vi "setfilter.vi"(2 "error in (no error)":errorcluster, 3 "Filter":i32=1 min=1 max=6 step=1) -> (0 "error out":errorcluster)   [LabVIEW 2017]
doc: "Selects the filter for monochromator to use"
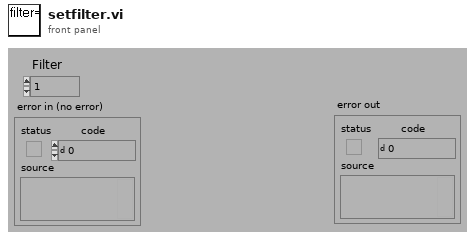
[diagram p1: front panel]
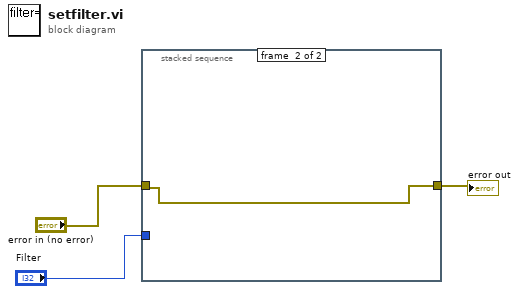
[diagram p0: block diagram]
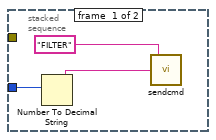
[diagram p2: hidden frame]
diagram:
  n1 = stacked-sequence {
    tunnel: "error in (no error)" -> [_ w7]
    tunnel: [_ w7] -> w2
    tunnel: "Filter" -> [w6 _]
    frame #0 {
      n2 = Number To Decimal String(number=w6) -> (decimal integer string=w4:string)  [unwired: 1 in]
      n3 = call "sendcmd.vi"("parameter"=w4, "command in"="FILTER") -> ()  [unwired: 1 in, 1 out]
    }
    frame #1 {
    }
  }
  "error out" <- w2
